vi "WhereHindbraintoMidbrainFilterCalibrate.vi"(3 "WhereAmI? Raw":T1) -> (1 "WhereAmI? Clean":T1)   [LabVIEW 2010]
doc: "This subVI takes raw I16 \"Where am I?\" data from the hindbrain and filters and calibrates it to become clean double data for the Midbrain. Cluster is:\n\nt=time\nx=horizontal position\ny=vetical position"
panel:
  # "This subVI filters and \nand calabrates the\nWhere am I? data \nfrom the hindbrain"
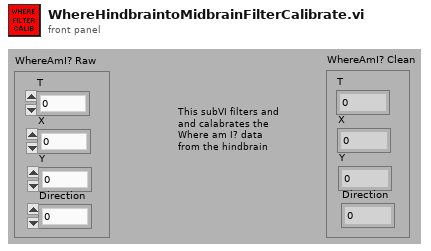
[diagram p1: front panel]
types:
  T1 = cluster{"T":dbl, "X":dbl, "Y":dbl, "Direction":dbl}
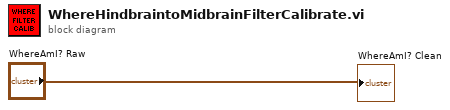
[diagram p0: block diagram]
diagram:
  "WhereAmI? Clean" <- "WhereAmI? Raw"
